vi "Check Subset (Power of 2).vi"(5 "power of 2":i16, 7 "source vi name":string, 8 "error in (no error)":errorcluster, 9 "offset (0)":u64 format="%08x bytes", 10 "count":u64 format="%08x bytes", 11 "Pointer in":refnum<class "Pointer.lvclass">) -> (0 "error out":errorcluster, 1 "offset out":u64 format="%08x bytes", 2 "count":u64 format="%08x bytes", 3 "Pointer out":refnum<class "Pointer.lvclass">)   [LabVIEW 2017, in "Memory Manager.lvlib" / "Pointer.lvclass"]
uses:
  Pointer.lvclass
  Pointer.lvclass/Pointer.ctl
  Error VIs/Out of Bounds.vi
  Error Building/Write Pointer Size.vi
  Error Building/Create Error.vi
  Error Building/Get Error Info.vi
  VIs/Write String into Source.vi
  VIs/Write Number into Source.vi
  VIs/VIs for Poly/Write U64 into Source.vi
  VIs/Set Error Source.vi
  VIs/Set Error Code.vi
  VIs/Set Error Status.vi
  Constants/Constants.vi
  Constants/Library Name.vi
  VIs/Create Error Cluster.vi
  VIs/VIs for Poly/Create Error Cluster (256B).vi
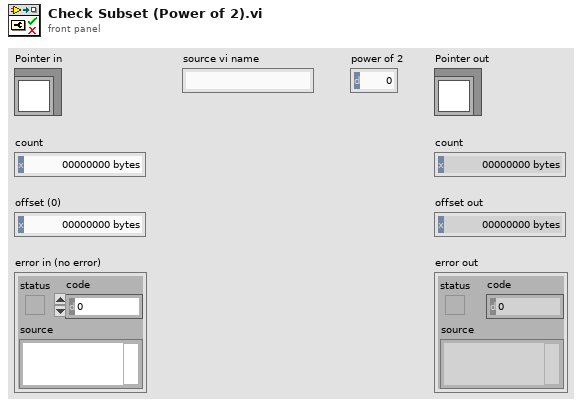
[diagram p1: front panel]
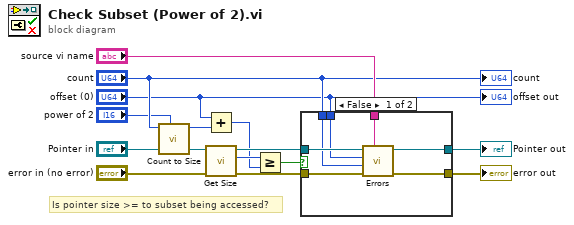
[diagram p0: block diagram]
diagram:
  # "Is pointer size >= to subset being accessed?"
  n1 = call "Count to Size.vi"("power of 2"="power of 2", "count"="count") -> ("size"=w4:u64)  [unwired: 9 in]
  n2 = Add(x="offset (0)", y=w4) -> (x+y=w2:u64)
  n3 = call "Get Size.vi"("Pointer in"="Pointer in") -> ("size"=w11:u64, "Pointer out"=w8:refnum<class "Pointer.lvclass">)  [unwired: 9 in]
  n4 = Greater Or Equal?(x=w11, y=w2) -> (x >= y?=w9:bool)
  n5 = case shown="False" w9 {
    tunnel: w8 -> [w20 w21]
    tunnel: "error in (no error)" -> [w18 w22]
    tunnel: [w17 w22] -> w13
    tunnel: [w19 w21] -> w12
    tunnel: "offset (0)" -> [w16 _]
    tunnel: "count" -> [w15 _]
    tunnel: "source vi name" -> [w14 _]
    frame False {
      n6 = call-poly "Errors.vi"("error source vi name"=w14, "error in (no error)"=w18, "length"=w15, "offset"=w16, "Pointer in"=w20) -> ("error out"=w17:errorcluster, "Pointer out"=w19:refnum<class "Pointer.lvclass">)  [unwired: 5 in]
    }
    frame True {
    }
  }
  "error out" <- w13
  "Pointer out" <- w12
  "offset out" <- "offset (0)"
  "count" <- "count"
